vi "all_on_normalizer.vi"(5 "CH 0 frequency":dbl[](array[numeric])=[20.35468, 23.0, 25.0, 25.0, 25.0, 25.0, 27.0, 27.0, 27.0, 24.0, 24.0, 24.0, 25.0, 25.0, 25.0, 25.0, 25.0, 25.0, 26.0, 26.0, 26.0, 26.0, 26.0, 26.0, 27.0, 27.0, 27.0, 27.0, 27.0, 27.0, 28.0, 28.0, 28.0, 28.0, 28.0, 28.0]) -> (1 "Normalized CH 0":dbl[](array[numeric])=[0.8560695599784639, 0.886297539, 0.892346939, 0.892346939, 0.892346939, 0.892346939, 0.916965996, 0.916965996, 0.916965996, 0.886297539, 0.886297539, 0.886297539, 0.892346939, 0.892346939, 0.892346939, 0.892346939, 0.892346939, 0.892346939, 0.889301802, 0.889301802, 0.889301802, 0.889301802, 0.889301802, 0.889301802, 0.916965996, 0.916965996, 0.916965996, 0.916965996, 0.916965996, 0.916965996, 0.939716312, 0.939716312, 0.939716312, 0.939716312, 0.939716312, 0.939716312])   [LabVIEW 2020]
uses:
  <vilib>/Utility/file.llb/Read From Spreadsheet File (DBL).vi
  <vilib>/gmath/NI_Gmath.lvlib
panel:
  in  "CH 0 Data Path (.csv)":path=path "C:/Users/yalem/Documents/Optlev/LabView Code/ARRAY/Power Normalization Files/sigpowernorm_9-2-23.csv"
  # "Makes sure that the power into the AOD is capped at 1.85W\nThis assumes that the attenuator is set at 6.9V"
  # "Power data for this normalization taken on:"
  # "Gives you the interpolated value to multiply the gain by to make sure the the high frequency signal does not overpower the aod and break it, while allowing higher power in the upper end of the aod range"
  # "Inputs:"
  # "Outputs:"
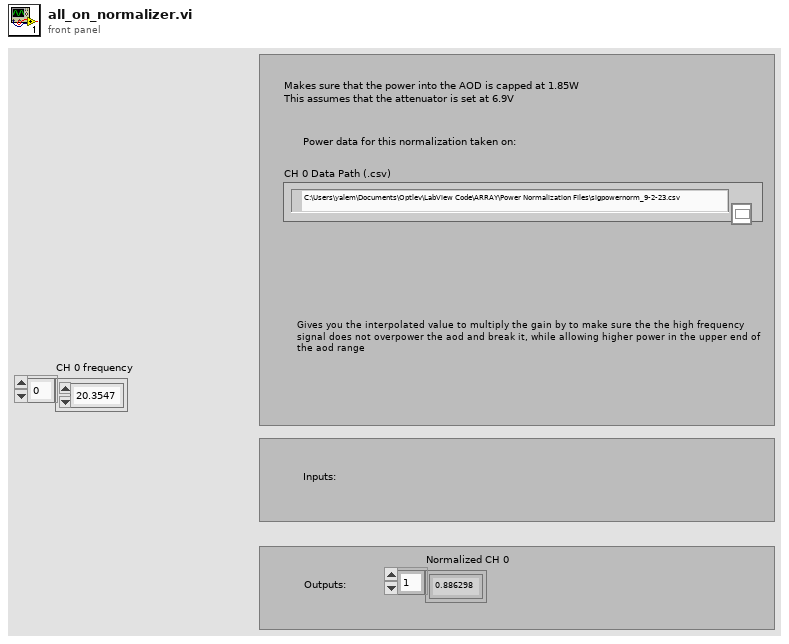
[diagram p1: front panel]
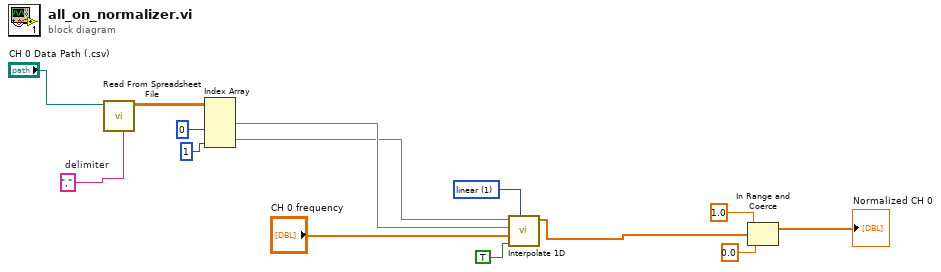
[diagram p0: block diagram]
diagram:
  w11 = 1 items=["nearest", "linear", "spline", "cubic Hermite", "Lagrange"] ("method")
  w14 = ","  # delimiter
  n1 = call-poly <vilib>:"Read From Spreadsheet File.vi"("delimiter (\\t)"=w14, "file path (dialog if empty)"="CH 0 Data Path (.csv)") -> ("all rows"=w13:dbl[][])  [unwired: 5 in, 4 out]
  n2 = Index Array(array=w13, index (col) #1=0, index (col) #2=1) -> (element #1=w9:dbl[], element #2=w8:dbl[])  [unwired: 2 in]
  n3 = call <vilib>:"Interpolate 1D.vi"("method"=w11, "X is monotonic"=TRUE, "xi"="CH 0 frequency", "X"=w9, "Y"=w8) -> ("yi"=w2:dbl[])  [unwired: 4 in, 2 out]
  n4 = In Range and Coerce(upper limit=1.0, x=w2, lower limit=0.0) -> (coerced(x)=→"Normalized CH 0":dbl[])  [unwired: 1 out]
